vi "Local Bus speed Test.vi"() -> ()   [LabVIEW 2021]
uses:
  <vilib>/TSA/Abstract Data Classes/Abs_Types/Double Float/Support/Type.ctl
  Source/Omni-Bus/Omni_Bus.lvclass
  Source/Local Bus/Local Bus.lvclass
  C:/Users/Tim/Documents/GitHub/Omni-Bus/Source/Omni-Bus/Bus Access/Bus_Access.lvclass
  <vilib>/Utility/Data Type/Type Definitions/Data Type.ctl
  Source/Omni-Bus/Bus Access/Bus_Access.lvclass/Bus_Access.ctl
  Source/Local Bus/Local Bus.lvclass/Local Bus.ctl
  Source/Omni-Bus/Bus Access/Properties/Write Tags.vi
  Source/Local Bus/Properties/Write Tag Types.vi
  <vilib>/TSA/Abstract Data Classes/Abs_Types/Double Float/Abs_Double Float.lvclass
  <vilib>/Utility/Data Type/NI_Data Type.lvlib
  C:/Program Files (x86)/National Instruments/LabVIEW 2021/vi.lib/TSA/Abstract Data Classes/Abs_Types/Type/Abs_Type.lvclass
  C:/Users/Tim/Documents/GitHub/Omni-Bus/Source/Local Bus/Local Bus.lvclass
panel:
  out "error out":errorcluster
  out "x-y":dbl format="%#_6p"
  out "Value":T1
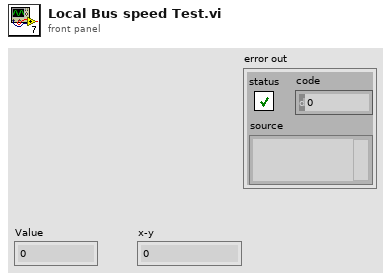
[diagram p1: front panel]
types:
  T1 = typedef "Abs_Double Float.lvclass/Type.ctl" = dbl
  T2 = typedef "NI_Data Type.lvlib/Data Type.ctl" = enum8{"Invalid Type", "Void", "I8", "I16", "I32", "I64", "U8", "U16", "U32", "U64", "Single Float", "Double Float", "Extended Float", "Single Complex", "Double Complex", "Extended Complex", "Enum U8", "Enum U16", "Enum U32", "Enum U64", "Single Float With Unit", "Double Float With Unit", "Extended Float With Unit", "Single Complex with Unit", "Double Complex with Unit", "Extended Complex with Unit", "Boolean", "String", "Path", "Picture", "Tag", "Array", "Cluster", "Variant", "LV Variant", "Waveform", "Timestamp", "Digital Waveform", "Digital Data", "ExpressData", "Refnum", "External Data", "VI", "Poly VI", "LabVIEW Class Instance", "Fixed Point", "Set Collection", "Map Collection"}
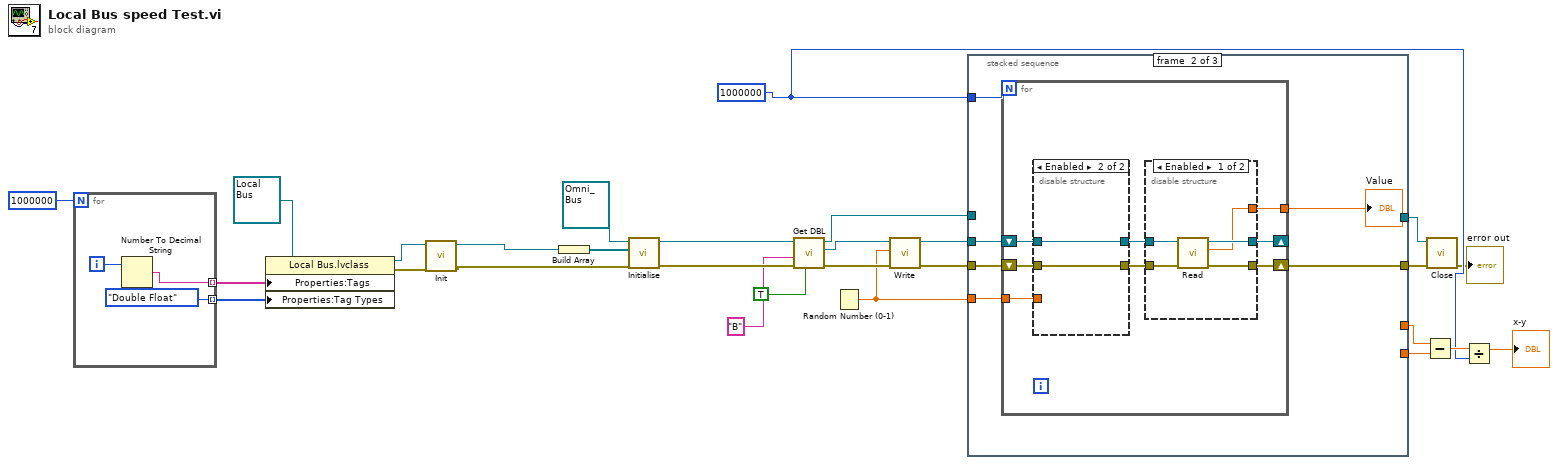
[diagram p0: block diagram]
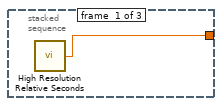
[diagram p2: hidden frame]
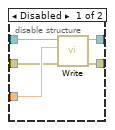
[diagram p3: hidden frame]
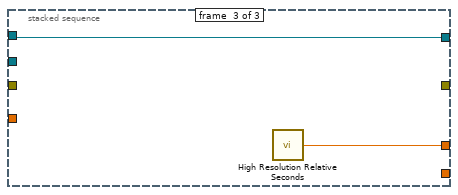
[diagram p5: hidden frame]
diagram:
  w19 = 1000000
  n1 = for {
    N: 1000000 -> [_]
    tunnel: [w30] -> w3 mode=indexing
    tunnel: [Data_Type."Double Float" ("Tag Type")] -> w2 mode=indexing
    i -> [w31]
    n2 = Number To Decimal String(number=w31) -> (decimal integer string=w30:string)  [unwired: 1 in]
  }
  n3 = property class="Local Bus.lvclass"(reference=refnum<class "Local Bus.lvclass"> refnum ("Local Bus.lvclass"), "Properties:Tags"=w3, "Properties:Tag Types"=w2) -> (reference out=w10:refnum<class "Local Bus.lvclass">, error out=w12:errorcluster)  [unwired: 1 in]
  n4 = call-dynamic "Init.vi"("error in (no error)"=w12, "Data in"=w10) -> ("error out"=w13:errorcluster, "Data out"=w14:refnum<class "Local Bus.lvclass">)  [unwired: 8 in]
  n5 = Build Array(w14) -> (w27:refnum<class "Local Bus.lvclass">[])
  n6 = call-dynamic "Initialise.vi"("error in (no error)"=w13, "Bus Access"=w27, "Var Bus in"=refnum<class "Omni_Bus.lvclass"> refnum) -> ("error out"=w25:errorcluster, "Var Bus out"=w26:refnum<class "Omni_Bus.lvclass">)  [unwired: 7 in]
  n7 = call-dynamic "Get DBL.vi"("Write?"=TRUE, "error in (no error)"=w25, "Tag"="B", "Var Bus in"=w26) -> ("error out"=w9:errorcluster, "Value Out"=w8:refnum<class "Abs_Double Float.lvclass">, "Var Bus out"=w16:refnum<class "Omni_Bus.lvclass">)  [unwired: 5 in]
  n8 = Random Number (0-1)() -> (number: 0 to 1=w5:dbl)
  n9 = call-dynamic "Write.vi"("error in (no error)"=w9, "Value"=w5, "Double Float.lvclass in"=w8) -> ("error out"=w6:errorcluster, "Double Float.lvclass out"=w7:refnum<class "Abs_Double Float.lvclass">)  [unwired: 7 in]
  n10 = stacked-sequence {
    tunnel: w7 -> [_ w36 _]
    tunnel: w6 -> [_ w35 _]
    tunnel: [_ _ w61] -> w24
    tunnel: [_ _ w62] -> w23
    tunnel: [w32 _ _] -> w22
    tunnel: w19 -> [_ w37 _]
    tunnel: w16 -> [_ _ w61]
    tunnel: [_ w34 _] -> w15
    tunnel: w5 -> [_ w33 _]
    frame #0 {
      n11 = call <vilib>:"High Resolution Relative Seconds.vi"() -> ("relative seconds"=w32:dbl)
    }
    frame #1 {
      n12 = for {
        N: w37 -> [_]
        shift-right: [w46] -> _
        shift-left: w36 -> [w40]
        tunnel: [w45] -> w38
        shift-right: [w44] -> w34
        shift-left: w35 -> [w39]
        tunnel: w33 -> [w41]
        n13 = disable-structure shown="Enabled" {
          disable-tunnel: [w48 w53] -> w43
          disable-tunnel: [w51 w52] -> w42
          disable-tunnel: w41 -> [w50 _]
          disable-tunnel: w40 -> [w49 w53]
          disable-tunnel: w39 -> [w47 w52]
          frame Disabled {
            n14 = call-dynamic "Write.vi"("error in (no error)"=w47, "Value"=w50, "Double Float.lvclass in"=w49) -> ("error out"=w51:errorcluster, "Double Float.lvclass out"=w48:refnum<class "Abs_Double Float.lvclass">)  [unwired: 7 in]
          }
          frame Enabled {
          }
        }
        n15 = disable-structure shown="Enabled" {
          disable-tunnel: [w58 w60] -> w46
          disable-tunnel: [w57 _] -> w45
          disable-tunnel: [w56 w59] -> w44
          disable-tunnel: w43 -> [w55 w60]
          disable-tunnel: w42 -> [w54 w59]
          frame Enabled {
            n16 = call-dynamic "Read.vi"("error in (no error)"=w54, "Double Float.lvclass_340760 in"=w55) -> ("error out"=w56:errorcluster, "Value"=w57:T1, "Double Float.lvclass_340760 out"=w58:refnum<class "Abs_Double Float.lvclass">)  [unwired: 7 in]
          }
          frame Disabled {
          }
        }
      }
      "Value" <- w38
    }
    frame #2 {
      n17 = call <vilib>:"High Resolution Relative Seconds.vi"() -> ("relative seconds"=w62:dbl)
    }
  }
  n18 = Subtract(x=w23, y=w22) -> (x-y=w21:dbl)
  n19 = call-dynamic "Close.vi"("error in (no error)"=w15, "Data in"=w24) -> ("error out"=→"error out":errorcluster)  [unwired: 8 in, 1 out]
  n20 = Divide(x=w21, y=w19) -> (x/y=→"x-y":dbl)
